vi "Radar_Wireless_Reception_Gating_read and write_multiplexer - Copy - Copy - Copy.vi"(0 "VISA resource name":refnum<visa-resource-name>="COM1", 1 "baud rate":u32=9600, 4 "data bits":u16=8 min=5 max=8 step=1, 5 "parity":u16(ring) items=["None", "Odd", "Even", "Mark", "Space"], 7 "stop bits":u16(ring)=10 items=["1.0"=10, "1.5"=15, "2.0"=20], 9 "XON Character":u8=17 format="%.0x", 14 "XOFF Character":u8=19 format="%.0x", 15 "timeout (ms)":u32=10000, 21 "End read on termination character?":bool=TRUE, 24 "termination char\n(0xA = '\\n' = LF)":u8=10 format="%.0x", 25 "Input\nbuffer size":u32=4096) -> ()   [LabVIEW 2012]
doc: "The Advanced Serial Read and Write example performs a Serial Port Read, a Serial Port Write, or a combination of these actions while setting some advanced serial features like buffer size, termination characters, and XON/XOFF flow control. The user selects the actions (read or write) on the front panel. If both are selected, the VI will write the data first, read the data and then close the VISA session that is opened to the port. \n\nThe parameters set for the serial port must match the parameters of the connected instrument or device. In this example, the bytes to read parameter specifies the number of bytes that the serial port reads. If there were more bytes at the port than the number specified in bytes to read, those bytes would not be read. Also, if you specify to read more bytes than the number of bytes actually read, you might receive a timeout error message.\n\nINSTRUCTIONS:\n1) Select the serial resource and configuration parameters (baud rate, data bits, parity, stop bits, flow control).\n2) Termination character can be enabled and set. Also, set the required input buffer size prior to running the example.\n3) Select the operations to be performed. \n4) Connect the serial port to your device. If no device is available, perform a loopback test by doing one of the following. Short pins 2 and 3 on a RS-232 cable or short pin 4 to pin 8 and pin 5 to pin 9 on a RS-485/422 cable. \n5) Run the VI to see the data read. (The \"read string\" will match the \"string to write\" if a loopback test was performed.)\n\nThis example exposes several advanced features that you may need for your application. Not all applications need all the features shown in this example. The input buffer size is likely an important setting that you want to control in your application. This example expands upon the flow control option for XON and XOFF, allowing the user to choose those control characters. The timeout parameter has been brought to the front panel so a user can specify the time period the VISA Read will wait for the number of bytes to read before timing out. Also, the user has several controls for the termination character, which is discussed later.\n\nNote that you can press the write and read buttons and change the bytes to read parameters on the fly, while the example is running. However, you must stop the example to change the other configuration parameters after the example has started running, and then run again.\n\nSet the I/O buffer size slightly higher the amount of data you expect to receive. This is very important for applications that don't use flow control, as you may lose characters if the receive buffer overflows.\n\nSetting the timeout period ensures that the operation returns with a timeout error if the operation cannot be performed in the specified time period. \n\nSome devices require a termination character in order to identify the end of command strings. Some devices send a termination character to signify the end of data to be read. \n\nThis example shows how you can end the Read operation once a termination character is detected in the buffer and/or append a termination character at the end of the Write data. To enable the Read to end on a termination character, use the VISA Configure Serial Port or use the VISA Properties Serial End Mode for Reads, Termination Character Enable, and Termination Character. To end the Write with a termination character, use the VISA Properties Serial End Mode for Writes, the Send End Enable, and Termination Character. In this example, the same termination character is used for both the Read and the Write. You can specify two different characters for your application, if desired.\n\nYour application may require specific characters for the XON/XOFF Flow Control. You can specify these characters with the VISA Properties Flow Control XOFF Character and Flow Control XON Character. Note that if the standard XON and XOFF characters are used, then decimal 17 and 19 are unavailable for data values. Remember that using flow control and setting an adequate buffer size allow you to prevent buffer overflows."
uses:
  <vilib>/Instr/_visa.llb/VISA Configure Serial Port (Instr).vi
  <vilib>/measure/madcrms.llb/Basic Averaged DC-RMS for 1 Chan.vi
  <vilib>/express/express analysis/Spectral/Block/exnSpectralBlock spectral measurements peak poly.vi
  <vilib>/express/express analysis/Spectral/Block/exnSpectralBlock spectral measurements peak DDT.vi
  <vilib>/express/express analysis/Spectral/XNode/ExpressSpectralMeasurementsBlockNode.xnode
  <vilib>/measure/NI_MAPro.lvlib
panel:
  out "I channel":i16(knob) scale=0.0..255.0
  out "Q channel":i16(knob) scale=0.0..255.0
  in  "I Channel":i16(c297)
  in  "Q Channel":i16(c297)
  in  "string to write 2":string="*IDN?\n"
  in  "I Channel":bool
  in  "Q Channel":bool
  in  "Operating\nFrequency\nSwitch":bool
  in  "Slide 2":u32(slide) scale=1.0..3.0
  in  "string to write":string="*IDN?\r\n"
  in  "write 2":bool=TRUE
  out "I/Q Spectrum":dynamicdata(graph)
  in  "Save Data":bool
  out "I/Q channels":dynamicdata(graph)
  in  "t0":timestamp=timestamp(3198752888.296 s since 1904-01-01)
  in  "FFT":i32=256
  in  "stop":bool
  in  "flow control":u16(ring) items=["None"=0, "XON/XOFF"=1, "RTS/CTS"=2, "DTR/DSR"=4]
  # "10 V"
  # "-10 V"
  # "0 V"
  # "10 V"
  # "-10 V"
  # "0 V"
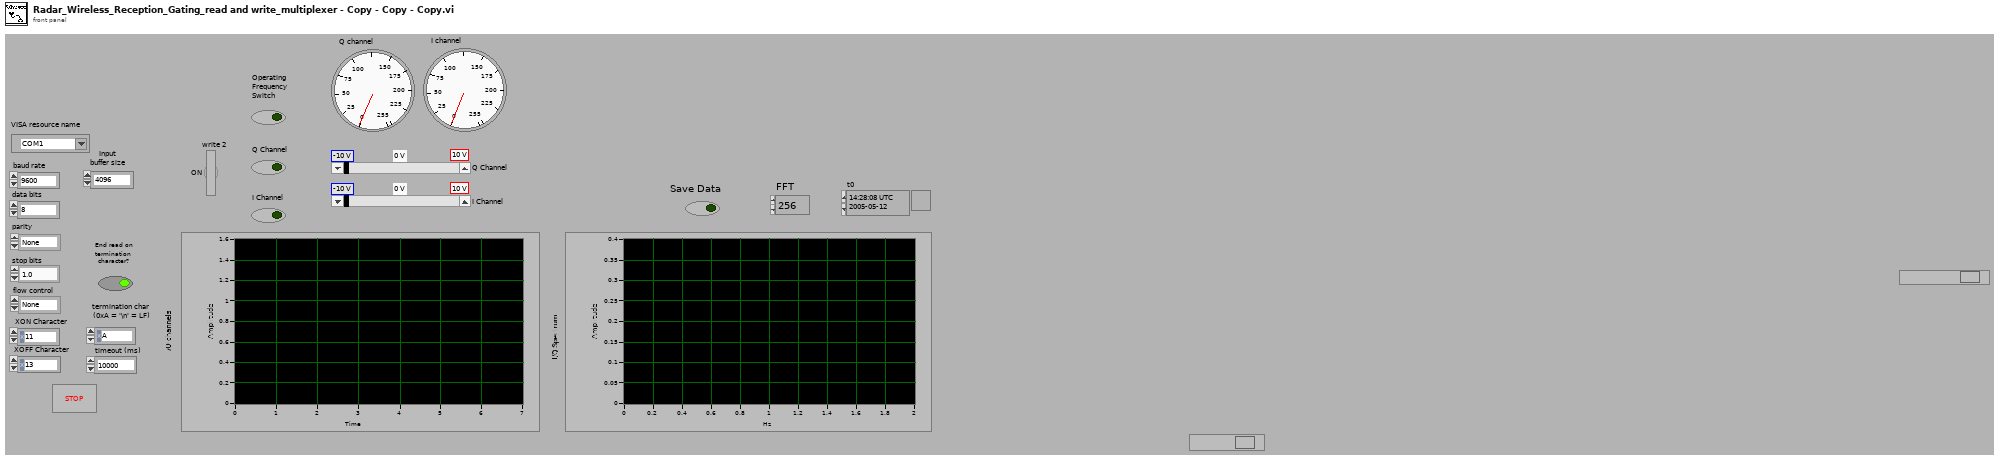
[diagram p1: front panel]
types:
  T1 = cluster{"averaging mode":u16, "weighting mode":u16, "number of averages":u32}
  T2 = cluster{"dB On (F)":bool, "unwrap phase (F)":bool, "convert to degree (F)":bool}
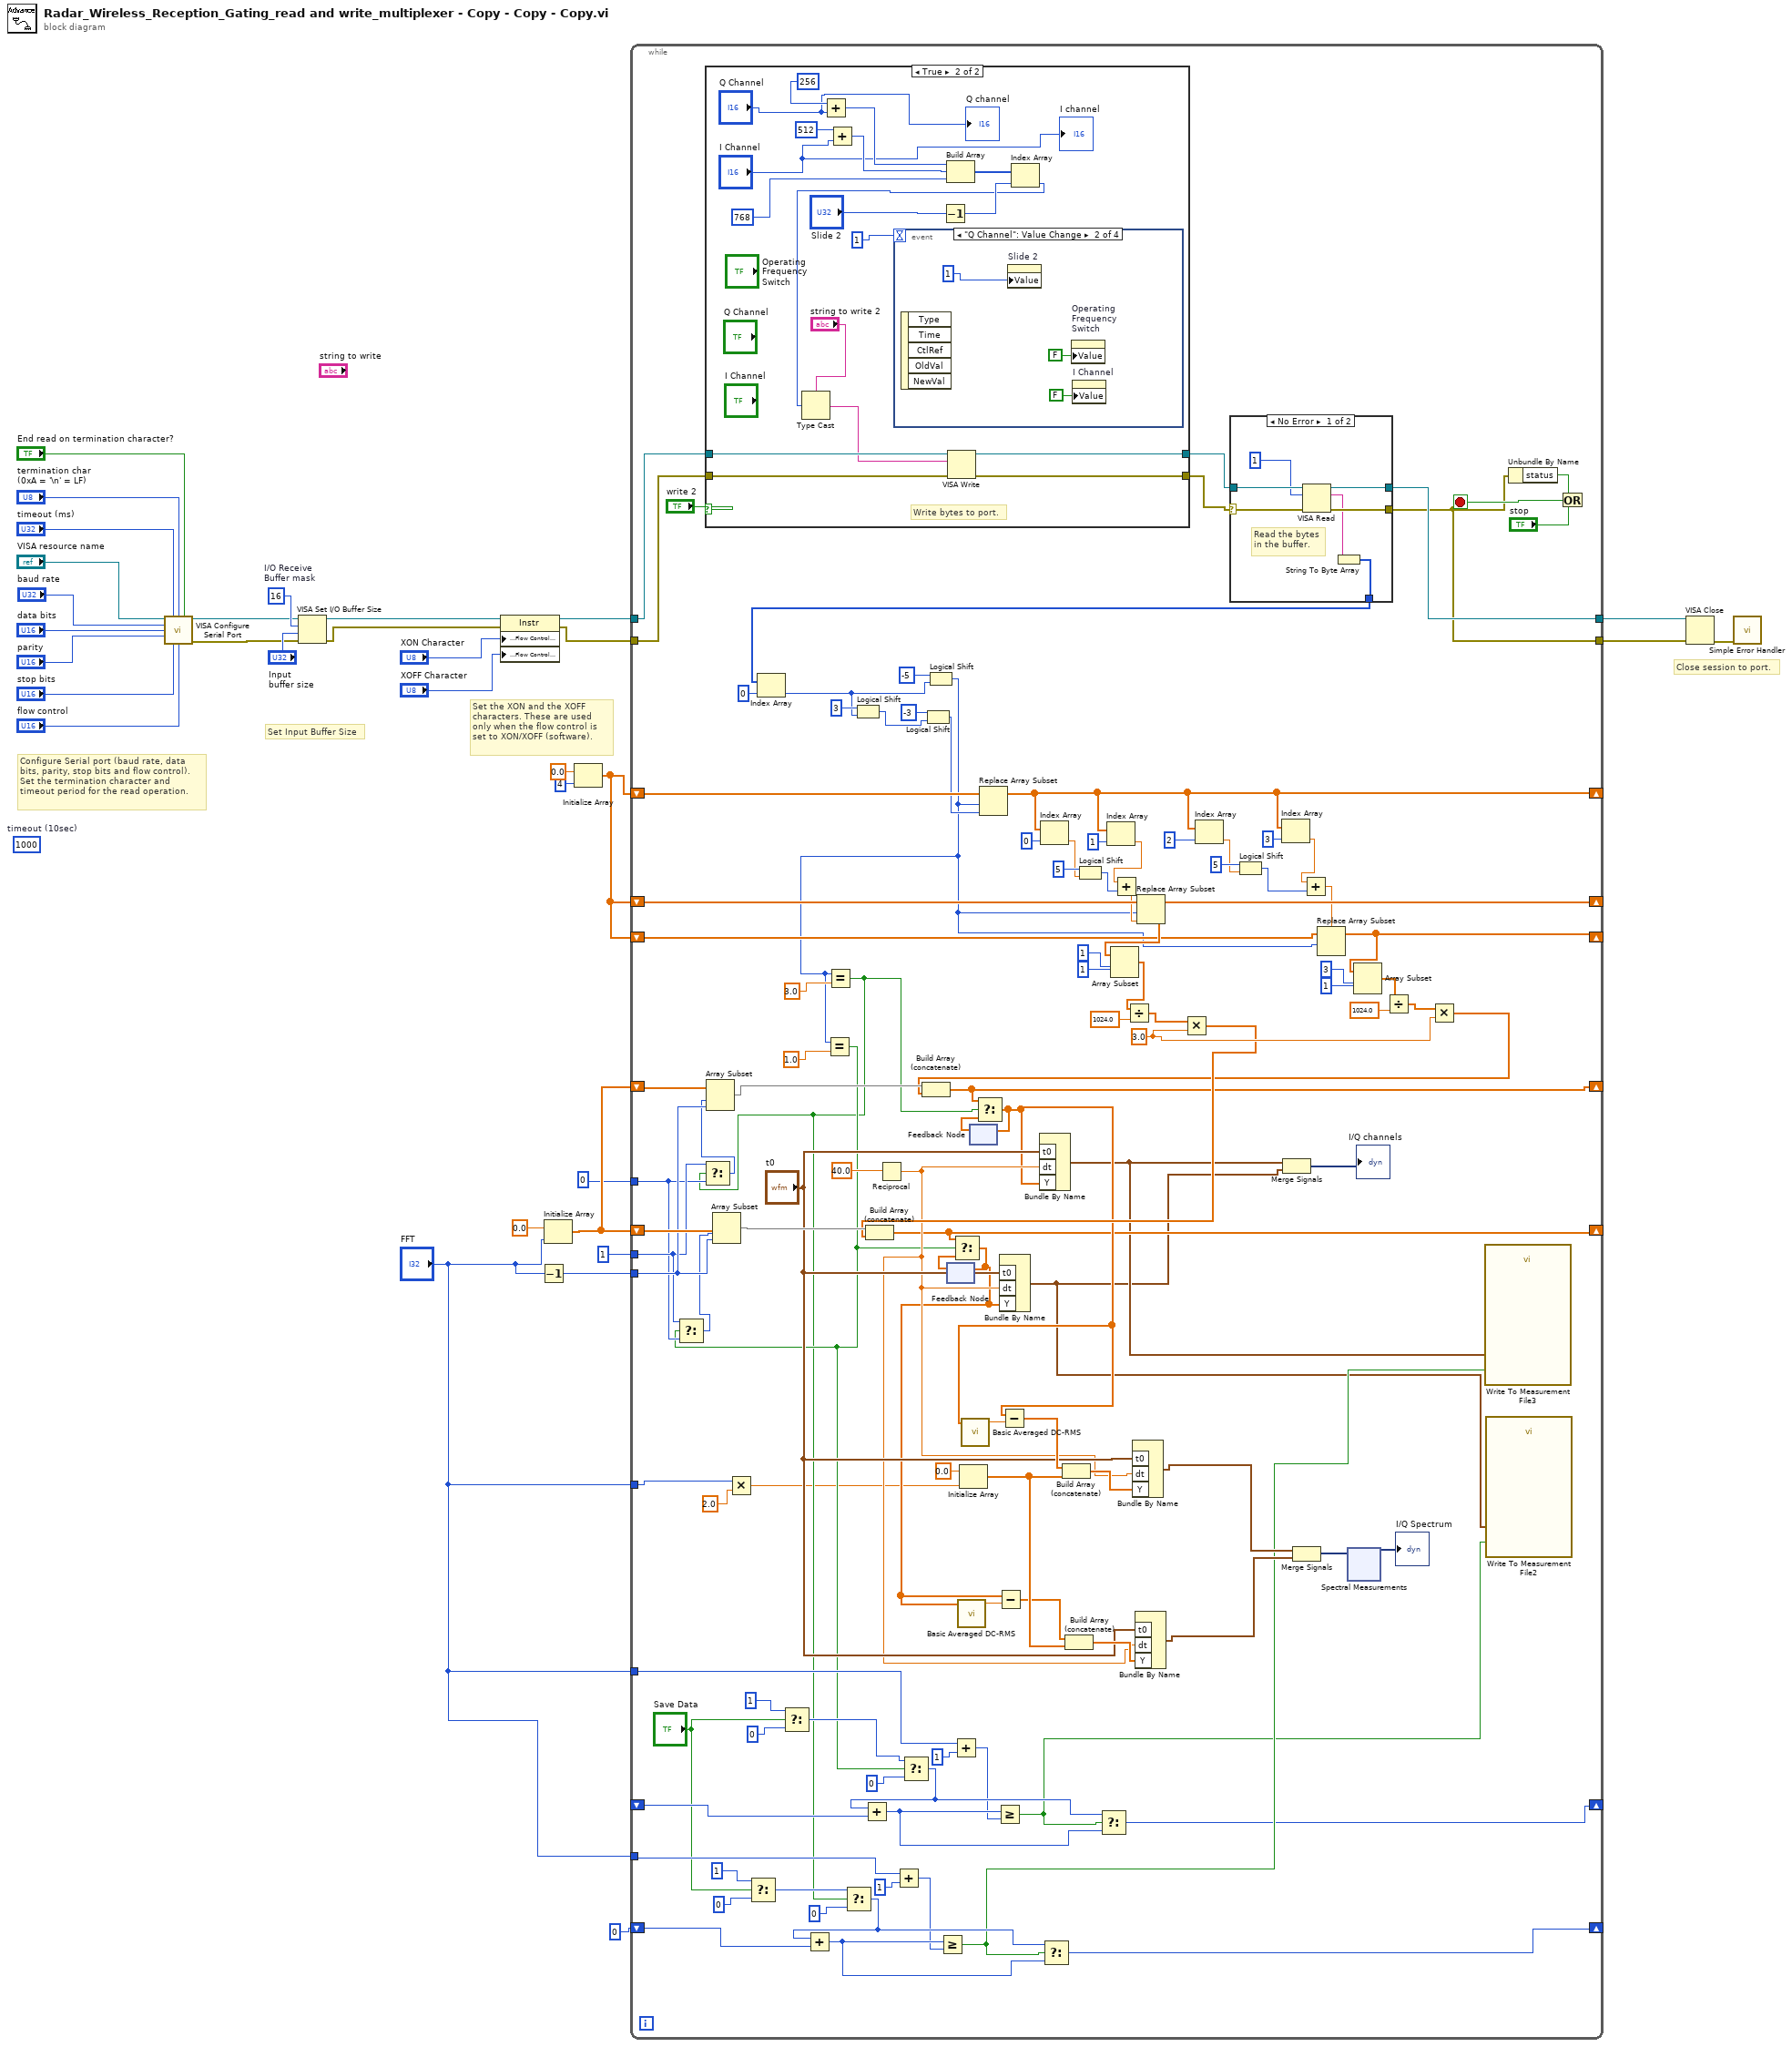
[diagram p0: block diagram]
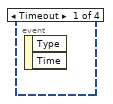
[diagram p3: hidden frame]
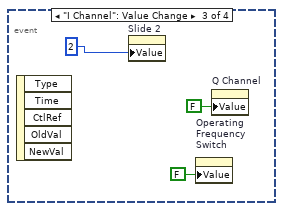
[diagram p4: hidden frame]
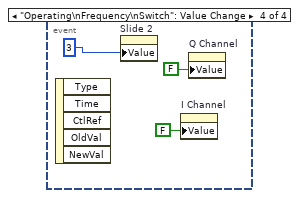
[diagram p5: hidden frame]
diagram:
  (unwired) u32 1000  # timeout (10sec)
  w25 = u16 16  # I/O Receive Buffer mask
  # "Set the XON and the XOFF\ncharacters. These are used\nonly when the flow control is\nset to XON/XOFF (software)."
  # "Configure Serial port (baud rate, data\nbits, parity, stop bits and flow control).\nSet the termination character and\ntimeout period for the read operation."
  # "Set Input Buffer Size"
  # "Close session to port."
  n1 = call-poly "VISA Configure Serial Port"("VISA resource name"="VISA resource name", "timeout (10sec)"="timeout (ms)", "termination char\n(0xA = '\\n' = LF)"="termination char\n(0xA = '\\n' = LF)", "Enable Termination\nChar (T)"="End read on termination character?", "baud rate (9600)"="baud rate", "data bits (8)"="data bits", "parity (0:none)"="parity", "stop bits (10: 1 bit)"="stop bits", "flow control (0:none)"="flow control") -> ("VISA resource name out"=w2:refnum<visa-resource-name>, "error out"=w1:errorcluster)  [unwired: 1 in, 4 out]
  n2 = VISA Set I/O Buffer Size(VISA resource name=w2, mask (16)=w25, size (4096)="Input\nbuffer size", error in (no error)=w1) -> (VISA resource name out=w21:refnum<visa-resource-name>, error out=w20:errorcluster)
  n3 = property class="Instr"(reference=w21, error in=w20, "Serial Settings:Flow Control XON Character"="XON Character", "Serial Settings:Flow Control XOFF Character"="XOFF Character") -> (reference out=w15:refnum<visa-resource-name>, error out=w17:errorcluster)
  n4 = Decrement(x="FFT") -> (x-1=w12:i32)
  n5 = Initialize Array(0.0 ("element"), "FFT") -> (w8:dbl[])
  n6 = Initialize Array(0.0 ("element"), 4 ("dimension size")) -> (w7:dbl[])
  n7 = while {
    tunnel: w17 -> [w35]
    tunnel: w15 -> [w36]
    tunnel: [w120] -> w14
    tunnel: [w119] -> w13
    tunnel: w12 -> [w121]
    tunnel: 1 ("index") -> [w65]
    shift-right: [w67] -> _
    shift-left: w8 -> [w144]
    shift-right: [w132] -> _
    shift-left: w7 -> [w138]
    shift-right: [w73] -> _
    shift-left: w8 -> [w122]
    shift-right: [w111] -> _
    shift-left: w7 -> [w113]
    shift-right: [w103] -> _
    shift-left: w7 -> [w106]
    shift-right: [w85] -> _
    shift-left: 0 -> [w88]
    tunnel: "FFT" -> [w81]
    tunnel: "FFT" -> [w39]
    tunnel: 0 ("index") -> [w64]
    tunnel: "FFT" -> [w54]
    shift-right: [w49] -> _
    shift-left: _ -> [w50]
    stop <- w148 stop-if-true
    (unwired) 0
    w93 = 3.0 ("y")
    n8 = case shown="True" "write 2" {
      tunnel: [w151 w166] -> w33
      tunnel: w36 -> [w150 w169]
      tunnel: w35 -> [w151 w168]
      tunnel: [w150 w167] -> w34
      frame False {
      }
      frame True {
        # "Write bytes to port."
        n9 = Add(x=i16 256, y="Q Channel") -> (x+y=w161:i16)
        n10 = Add(x=i16 512, y="I Channel") -> (x+y=w157:i16)
        n11 = event shown="[1] \"Q Channel\": Value Change" {
          selector: _ -> [_ _ _ _]
          dyn-events: _ -> [_ _ _ _]
          timeout: i16 1 ("delay before read (ms)") -> [_ _ _ _]
          event Timeout {
            n12 = event-data() -> ()  [unwired: 1 in, 2 out]
          }
          event "Q Channel": Value Change {
            n13 = event-data() -> ()  [unwired: 1 in, 5 out]
            n14 = property on="Slide 2" class="Slide (strict)"("Value"=i16 1 ("delay before read (ms)")) -> ()  [unwired: 2 in, 2 out]
            n15 = property on="Operating\nFrequency\nSwitch" class="Bool (strict)"("Value"=FALSE ("Boolean 3")) -> ()  [unwired: 2 in, 2 out]
            n16 = property on="I Channel" class="Bool (strict)"("Value"=FALSE ("Boolean 2")) -> ()  [unwired: 2 in, 2 out]
          }
          event "I Channel": Value Change {
            n17 = event-data() -> ()  [unwired: 1 in, 5 out]
            n18 = property on="Slide 2" class="Slide (strict)"("Value"=i16 2 ("delay before read (ms)")) -> ()  [unwired: 2 in, 2 out]
            n19 = property on="Operating\nFrequency\nSwitch" class="Bool (strict)"("Value"=FALSE ("Boolean 3")) -> ()  [unwired: 2 in, 2 out]
            n20 = property on="Q Channel" class="Bool (strict)"("Value"=FALSE ("Boolean")) -> ()  [unwired: 2 in, 2 out]
          }
          event "Operating\nFrequency\nSwitch": Value Change {
            n21 = event-data() -> ()  [unwired: 1 in, 5 out]
            n22 = property on="Slide 2" class="Slide (strict)"("Value"=i16 3 ("delay before read (ms)")) -> ()  [unwired: 2 in, 2 out]
            n23 = property on="I Channel" class="Bool (strict)"("Value"=FALSE ("Boolean 2")) -> ()  [unwired: 2 in, 2 out]
            n24 = property on="Q Channel" class="Bool (strict)"("Value"=FALSE ("Boolean")) -> ()  [unwired: 2 in, 2 out]
          }
        }
        n25 = Decrement(x="Slide 2") -> (x-1=w163:u32)
        n26 = Build Array(w161, w157, i16 768 ("delay before read (ms)")) -> (w164:i16[])
        n27 = Index Array(array=w164, index=w163) -> (element=w156:i16)
        n28 = Type Cast(type="string to write 2", x=w156) -> (*(type *) &x=w154:string)
        n29 = VISA Write(VISA resource name=w169, write buffer=w154, error in (no error)=w168) -> (VISA resource name out=w167:refnum<visa-resource-name>, error out=w166:errorcluster)  [unwired: 1 out]
        "Q channel" <- "Q Channel"
        "I channel" <- "I Channel"
      }
    }
    n30 = Multiply(x=w39, y=2.0 ("dt")) -> (x*y=w40:dbl)
    n31 = Select(t=1, s="Save Data", f=0) -> (s? t:f=w51:i32)
    n32 = Select(t=1, s="Save Data", f=0) -> (s? t:f=w61:i32)
    n33 = Reciprocal(x=40.0 ("dt")) -> (1/x=w76:dbl)
    n34 = Add(x=w81, y=1) -> (x+y=w82:i32)
    n35 = feedback #1() -> (w69:dbl[])  [unwired: 1 out]
    n36 = Add(x=w54, y=1) -> (x+y=w55:i32)
    n37 = Initialize Array(0.0 ("element"), w40) -> (w97:dbl[])
    n38 = feedback #2() -> (w75:dbl[])  [unwired: 1 out]
    n39 = case "Read bytes from port." shown="No Error" w33 {
      selector: w33 -> [w193 w198]
      tunnel: [w195 w198] -> w119
      tunnel: [w196 w199] -> w120
      tunnel: w34 -> [w194 w199]
      tunnel: [w191 u8[] [] ("unsigned byte array")] -> w118
      frame No Error {
        # "Read the bytes\nin the buffer."
        n40 = VISA Read(VISA resource name=w194, byte count=u32 1, error in (no error)=w193) -> (VISA resource name out=w196:refnum<visa-resource-name>, read buffer=w192:string, error out=w195:errorcluster)  [unwired: 1 out]
        n41 = String To Byte Array(string=w192) -> (unsigned byte array=w191:u8[])
      }
      frame Error {
        # "Error occurred \nreading Bytes at \nSerial Port"
      }
    }
    n42 = Index Array(array=w118, index=0) -> (element=w141:u8)
    n43 = Logical Shift(y=i8 3, x=w141) -> (x << y=w140:u8)
    n44 = Logical Shift(y=i8 -3, x=w140) -> (x << y=w137:u8)
    n45 = Logical Shift(y=i8 -5, x=w141) -> (x << y=w70:u8)
    n46 = Equal?(x=w70, y=1.0) -> (x = y?=w44:bool)
    n47 = Select(t=w65, s=w44, f=w64) -> (s? t:f=w63:i32)
    n48 = Array Subset(array=w144, index=w63, length=w121) -> (w146:dbl[])
    n49 = Equal?(x=w70, y=3.0) -> (x = y?=w43:bool)
    n50 = Select(t=w65, s=w43, f=w64) -> (s? t:f=w66:i32)
    n51 = Array Subset(array=w122, index=w66, length=w121) -> (w123:dbl[])
    n52 = Select(t=w51, s=w43, f=0) -> (s? t:f=w87:i32)
    n53 = Add(x=w87, y=w88) -> (x+y=w86:i32)
    n54 = Select(t=w61, s=w44, f=0) -> (s? t:f=w62:i32)
    n55 = Add(x=w62, y=w50) -> (x+y=w57:i32)
    n56 = Greater Or Equal?(x=w86, y=w82) -> (x >= y?=w84:bool)
    n57 = Replace Array Subset(array=w138, new element=w137, index=w70) -> (w132:dbl[])
    n58 = Greater Or Equal?(x=w57, y=w55) -> (x >= y?=w45:bool)
    n59 = Index Array(array=w132, index=0) -> (element=w130:dbl)
    n60 = Select(t=w87, s=w84, f=w86) -> (s? t:f=w85:i32)
    n61 = Logical Shift(y=i16 5, x=w130) -> (x << y=w126:u32)
    n62 = Select(t=w62, s=w45, f=w57) -> (s? t:f=w49:i32)
    n63 = Index Array(array=w132, index=1) -> (element=w127:dbl)
    n64 = Add(x=w127, y=w126) -> (x+y=w112:dbl)
    n65 = Replace Array Subset(array=w113, new element=w112, index=w70) -> (w111:dbl[])
    n66 = Array Subset(array=w111, index=1, length=1) -> (w108:dbl[])
    n67 = Divide(x=w108, y=1024.0) -> (x/y=w116:dbl[])
    n68 = Multiply(x=w116, y=w93) -> (x*y=w79:dbl[])
    n69 = Build Array (concatenate)(w146, w79) -> (w67:dbl[])
    n70 = Select(t=w67, s=w44, f=w69) -> (s? t:f=w68:dbl[])
    n71 = feedback-in #1(w68) -> ()
    n72 = call-poly <vilib>:"Basic Averaged DC-RMS.vi"("signal in"=w68) -> ("DC value"=w96:dbl)  [unwired: 4 in, 6 out]
    n73 = Subtract(x=w68, y=w96) -> (x-y=w95:dbl[])
    n74 = Bundle By Name("t0"="t0", "dt"=w76, "Y"=w68) -> (w46:waveform(dbl))  [unwired: 1 out]
    n75 = Build Array (concatenate)(w95, w97) -> (w98:dbl[])
    n76 = Bundle By Name("t0"="t0", "dt"=w76, "Y"=w98) -> (w90:waveform(dbl))  [unwired: 1 out]
    n77 = Index Array(array=w132, index=2) -> (element=w128:dbl)
    n78 = Logical Shift(y=i16 5, x=w128) -> (x << y=w124:u32)
    n79 = Index Array(array=w132, index=3) -> (element=w125:dbl)
    n80 = Add(x=w125, y=w124) -> (x+y=w107:dbl)
    n81 = Replace Array Subset(array=w106, new element=w107, index=w70) -> (w103:dbl[])
    n82 = Array Subset(array=w103, index=3, length=1) -> (w102:dbl[])
    n83 = Divide(x=w102, y=1024.0) -> (x/y=w114:dbl[])
    n84 = Multiply(x=w114, y=w93) -> (x*y=w78:dbl[])
    n85 = Build Array (concatenate)(w123, w78) -> (w73:dbl[])
    n86 = Select(t=w73, s=w43, f=w75) -> (s? t:f=w74:dbl[])
    n87 = call-poly <vilib>:"Basic Averaged DC-RMS.vi"("signal in"=w74) -> ("DC value"=w100:dbl)  [unwired: 4 in, 6 out]
    n88 = feedback-in #2(w74) -> ()
    n89 = Subtract(x=w74, y=w100) -> (x-y=w99:dbl[])
    n90 = Bundle By Name("t0"="t0", "dt"=w76, "Y"=w74) -> (w47:waveform(dbl))  [unwired: 1 out]
    n91 = Build Array (concatenate)(w99, w97) -> (w92:dbl[])
    n92 = Bundle By Name("t0"="t0", "dt"=w76, "Y"=w92) -> (w91:waveform(dbl))  [unwired: 1 out]
    n93 = Merge Signals(w47, w46) -> (→"I/Q channels":dynamicdata)
    n94 = Merge Signals(w91, w90) -> (w41:dynamicdata)
    n95 = xnode "Spectral Measurements"("Signals"=w41) -> ("FFT - (Peak)"=→"I/Q Spectrum":dynamicdata)  [unwired: 2 in, 3 out]
    n96 = call "Write To Measurement File3"("Signals"=w47, "Enable"=w84) -> ()  [unwired: 15 in, 3 out]
    n97 = call "Write To Measurement File2"("Signals"=w46, "Enable"=w45) -> ()  [unwired: 15 in, 3 out]
    n98 = Unbundle By Name(w119) -> ("status"=w149:bool)
    n99 = Or(x=w149, y="stop") -> (x .or. y?=w148:bool)
  }
  n100 = VISA Close(VISA resource name=w14, error in (no error)=w13) -> (error out=w30:errorcluster)
  n101 = call <vilib>:"Simple Error Handler.vi"("error in (no error)"=w30) -> ()  [unwired: 1 in, 8 out]
